vi "Send Response.vi"(0 "reference in":refnum<class "NS slave.lvclass">, 1 "response":string, 2 "data":variant, 5 "error in (no error)":errorcluster) -> (14 "reference out":refnum<class "NS slave.lvclass">, 19 "error out":errorcluster)   [LabVIEW 2019, in "CommandResponse communication.lvlib" / "NS slave.lvclass"]
doc: "Sends response message to master. Should be called after recieving and processing command"
uses:
  NS slave.lvclass
  C:/Barkhausen mmWave radar/Development/LV/Barkhausen mmWave hardware control/Host/Intertarget communication/CR slave_class/CR slave.lvclass
  <vilib>/Utility/error.llb/DialogType.ctl
  Error response.ctl
  ITC response.ctl
  CommandResponse communication.lvlib
  <vilib>/addons/_JKI.lib/Serialization/JSON/JKI JSON Serialization.lvlib
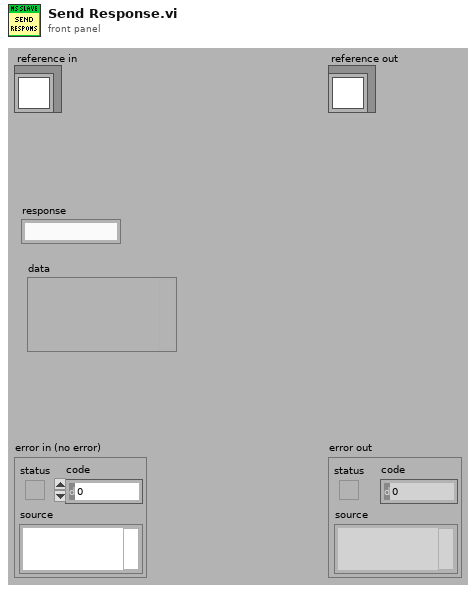
[diagram p1: front panel]
types:
  T1 = typedef "CommandResponse communication.lvlib/Error response.ctl" = cluster{"code":i32, "message":string, "source":string}
  T2 = typedef "DialogType.ctl" = u16
  T3 = typedef "CommandResponse communication.lvlib/NS slave.lvclass/ObjectAttributesRef.ctl" = refnum<data-value>
  T4 = typedef "CommandResponse communication.lvlib/ITC response.ctl" = cluster{"status":string, "reponse":string, "data":variant}
  T5 = typedef "CommandResponse communication.lvlib/NS slave.lvclass/ObjectAttributes.ctl" = cluster{"connected":bool, "stop":bool, "ID":string, "command rd":refnum<k21>, "response wr":refnum<k21>, "data wr":refnum<k21>}
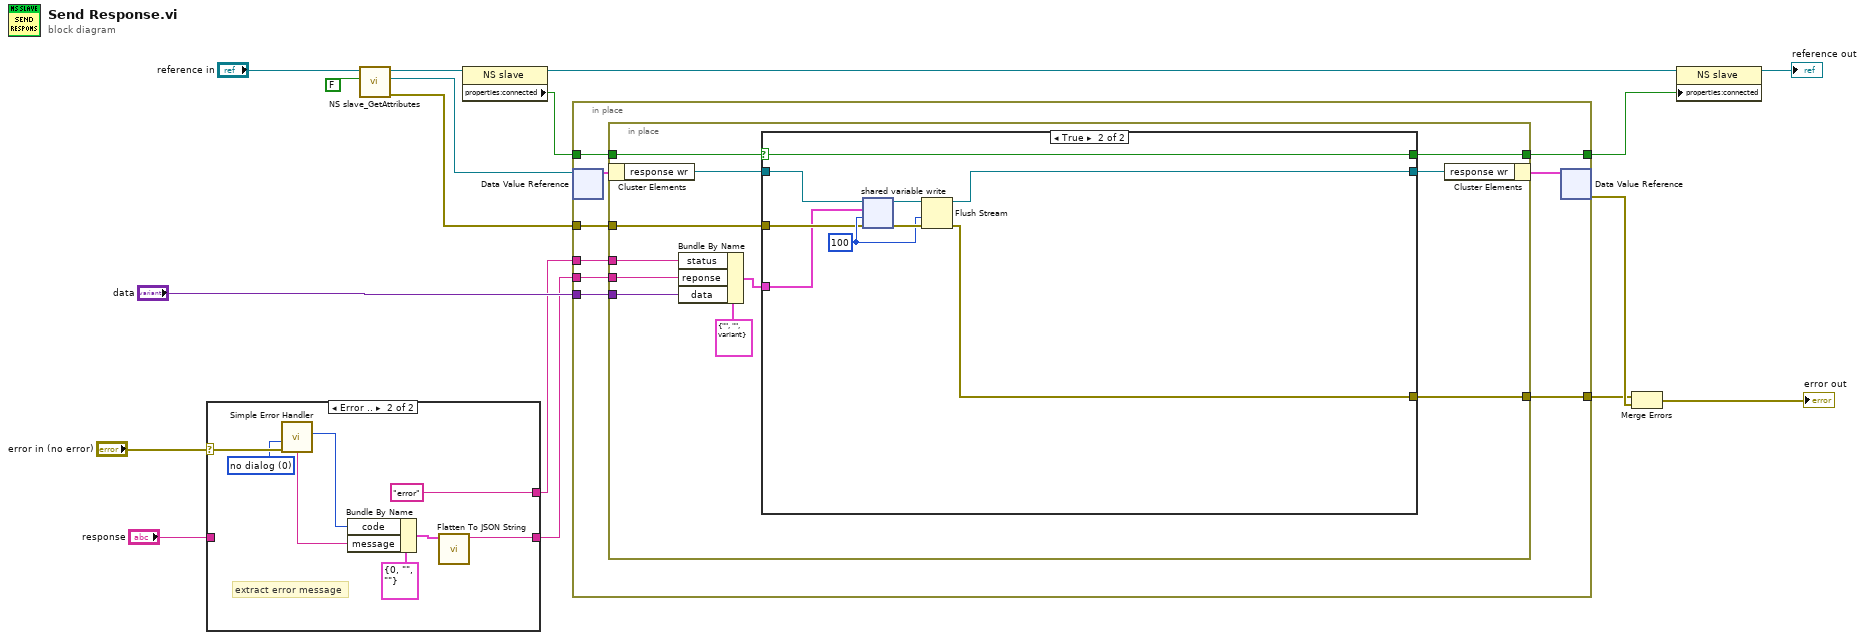
[diagram p0: block diagram]
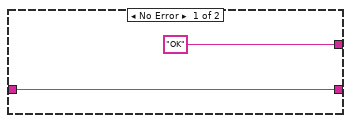
[diagram p2: hidden frame]
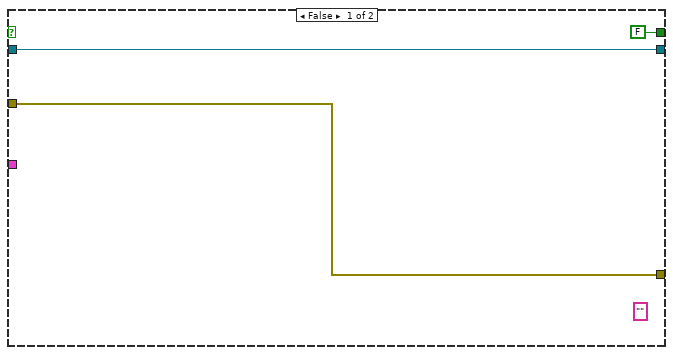
[diagram p3: hidden frame]
diagram:
  n1 = case shown="Error .." "error in (no error)" {
    selector: "error in (no error)" -> [_ w26]
    tunnel: ["OK" ("message") "error" ("message")] -> w3
    tunnel: [w18 w20] -> w2
    tunnel: "response" -> [w18 _]
    frame No Error {
    }
    frame Error {
      w25 = T2 0 items=["no dialog", "OK message", "continue or stop message", "OK message + warnings", "continue/stop + warnings"] ("type of dialog (OK msg:1)")
      # "extract error message"
      n2 = call <vilib>:"Simple Error Handler.vi"("type of dialog (OK msg:1)"=w25, "error in (no error)"=w26) -> ("code out"=w23:i32, "message"=w22:string)  [unwired: 3 in, 3 out]
      n3 = Bundle By Name(cluster=T1 {"code"=0, "message"="", "source"=""} ("Error response"), "code"=w23, "message"=w22) -> (w21:T1)
      n4 = call <vilib>:"Flatten To JSON String.vi"("Variant"=w21) -> ("JSON String"=w20:string)  [unwired: 9 in, 1 out]
    }
  }
  n5 = call "NS slave_GetAttributes.vi"("return data? (T)"=FALSE, "reference in"="reference in") -> ("error out"=w10:errorcluster, "attributes ref"=w11:T3, "reference out"=w15:refnum<class "NS slave.lvclass">)  [unwired: 6 in, 1 out]
  n6 = property class="NS slave"(reference=w15) -> (reference out=w8:refnum<class "NS slave.lvclass">, "properties:connected"=w7:bool)  [unwired: 1 in, 1 out]
  n7 = in-place {
    in-place-border: [w32] -> w13
    in-place-border: w2 -> [w34]
    in-place-border: w10 -> [w33]
    in-place-border: w3 -> [w31]
    in-place-border: "data" -> [w30]
    in-place-border: w7 -> [w29]
    in-place-border: [w28] -> w5
    n8 = in-place-dvr #1(w11) -> (w35:T5)  [unwired: 1 out]
    n9 = in-place {
      in-place-border: w34 -> [w44]
      in-place-border: w33 -> [w43]
      in-place-border: [w42] -> w32
      in-place-border: w31 -> [w40]
      in-place-border: w30 -> [w39]
      in-place-border: w29 -> [w38]
      in-place-border: [w37] -> w28
      n10 = in-place-cluster #2(w35) -> ("response wr"=w47:refnum<k21>)
      n11 = Bundle By Name(cluster=T4 {"status"="", "reponse"="", "data"=variant(cluster{"Boolean Round":bool, "code":i32, "source":string} {"Boolean Round"=FALSE, "code"=0, "source"=""})} ("data in"), "status"=w40, "reponse"=w44, "data"=w39) -> (w45:T4)
      n12 = case shown="True" w38 {
        selector: w38 -> [_ w52]
        tunnel: w47 -> [w50 w57]
        tunnel: [w50 w56] -> w46
        tunnel: w45 -> [_ w51]
        tunnel: w43 -> [w49 w53]
        tunnel: [w49 w54] -> w42
        tunnel: [FALSE w52] -> w37
        frame False {
          (unwired) "" ("reponse str")
        }
        frame True {
          w55 = 100 ("timeout ms (-1)")
          n13 = shared-variable-write(w57, w53, w51, w55) -> (w59:refnum<k21>, w58:errorcluster)  [unwired: 1 out]
          n14 = Flush Stream(8:w58, 9:w55, 11:w59) -> (0:w54:errorcluster, 3:w56:refnum<k21>)  [unwired: 1 in, 1 out]
        }
      }
      n15 = in-place-cluster #2("response wr"=w46) -> (w36:T5)
    }
    n16 = in-place-dvr #1(w36) -> (w14:errorcluster)  [unwired: 1 out]
  }
  n17 = Merge Errors(w13, w14) -> (→"error out":errorcluster)
  n18 = property class="NS slave"(reference=w8, "properties:connected"=w5) -> (reference out=→"reference out":refnum<class "NS slave.lvclass">)  [unwired: 1 in, 1 out]
